vi "Test Read Speed.vi"(8 "error in (no error)":errorcluster) -> (0 "error out":errorcluster)   [LabVIEW 2016]
uses:
  LV to ITX/LV to ITX.lvclass
panel:
  in  "length":i32=250
  out "Numeric 3":i32
  out "Numeric 2":i32
  out "Numeric":i32
  out "read TDMS (ms/file)":u32
  out "read HDF5 (ms/file)":u32
  out "read ITX (ms/file)":u32
  in  "TDMS Path":path
  in  "HDF5 Path":path
  in  "ITX Path":path
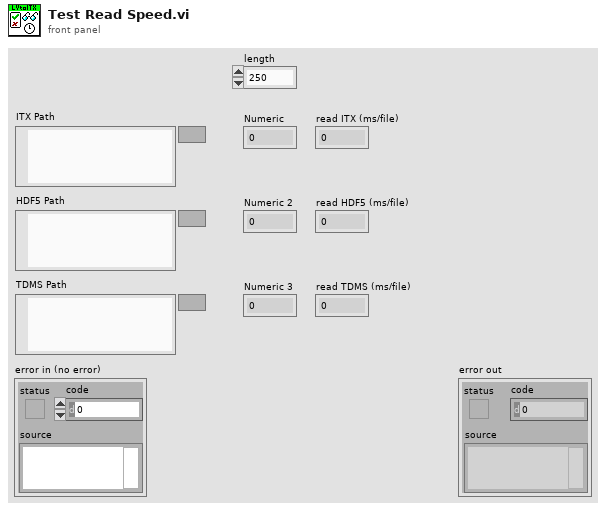
[diagram p1: front panel]
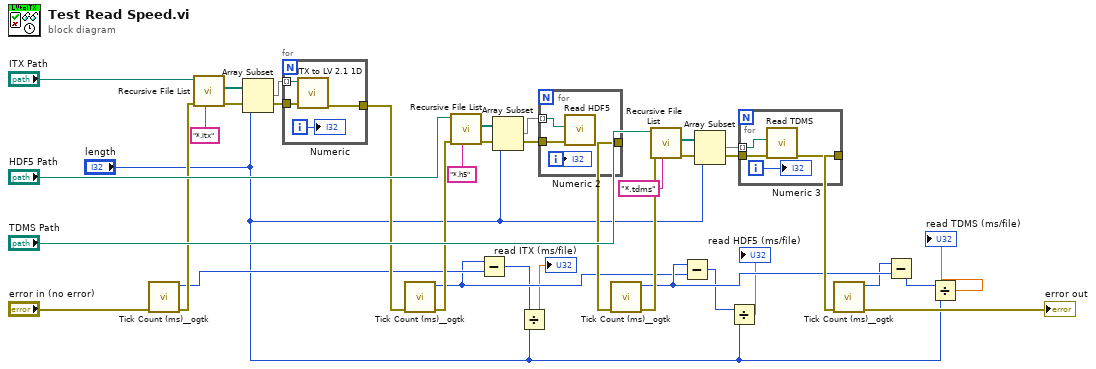
[diagram p0: block diagram]
diagram:
  n1 = call <userlib>:"Tick Count (ms)__ogtk.vi"("error in (no error)"="error in (no error)") -> ("error out"=w26:errorcluster, "millisecond timer value"=w15:u32)  [unwired: 9 in]
  n2 = call <vilib>:"Recursive File List.vi"("pattern"="*.itx", "error in (no error)"=w26, "Folder Path"="ITX Path") -> ("error out"=w9:errorcluster, "All Files in Dir"=w12:path[])  [unwired: 4 in, 3 out]
  n3 = Array Subset(array=w12, length="length") -> (w10:path[])  [unwired: 1 in]
  n4 = for {
    tunnel: w10 -> [w38] mode=indexing
    tunnel: [w37] -> w22
    tunnel: w9 -> [w36]
    i -> [w35]
    n5 = call "ITX to LV 2.1 1D.vi"("error in"=w36, "file (use dialog)"=w38) -> ("error out"=w37:errorcluster)  [unwired: 4 in, 5 out]
    "Numeric" <- w35
  }
  n6 = call <userlib>:"Tick Count (ms)__ogtk.vi"("error in (no error)"=w22) -> ("error out"=w21:errorcluster, "millisecond timer value"=w8:u32)  [unwired: 9 in]
  n7 = call <vilib>:"Recursive File List.vi"("pattern"="*.h5", "error in (no error)"=w21, "Folder Path"="HDF5 Path") -> ("error out"=w20:errorcluster, "All Files in Dir"=w29:path[])  [unwired: 4 in, 3 out]
  n8 = Subtract(x=w8, y=w15) -> (x-y=w7:u32)
  n9 = Array Subset(array=w29, length="length") -> (w24:path[])  [unwired: 1 in]
  n10 = Divide(x=w7, y="length") -> (x/y=→"read ITX (ms/file)":dbl)
  n11 = for {
    tunnel: w24 -> [w39] mode=indexing
    tunnel: w20 -> [w42]
    tunnel: [w41] -> w19
    i -> [w40]
    n12 = call "Read HDF5.vi"("error in (no error)"=w42, "path"=w39) -> ("error out"=w41:errorcluster)  [unwired: 4 in, 5 out]
    "Numeric 2" <- w40
  }
  n13 = call <userlib>:"Tick Count (ms)__ogtk.vi"("error in (no error)"=w19) -> ("error out"=w18:errorcluster, "millisecond timer value"=w14:u32)  [unwired: 9 in]
  n14 = call <vilib>:"Recursive File List.vi"("pattern"="*.tdms", "error in (no error)"=w18, "Folder Path"="TDMS Path") -> ("error out"=w17:errorcluster, "All Files in Dir"=w28:path[])  [unwired: 4 in, 3 out]
  n15 = Subtract(x=w14, y=w8) -> (x-y=w5:u32)
  n16 = Array Subset(array=w28, length="length") -> (w23:path[])  [unwired: 1 in]
  n17 = Divide(x=w5, y="length") -> (x/y=→"read HDF5 (ms/file)":dbl)
  n18 = for {
    tunnel: w23 -> [w46] mode=indexing
    tunnel: w17 -> [w45]
    tunnel: [w44] -> w16
    i -> [w43]
    n19 = call "Read TDMS.vi"("error in (no error)"=w45, "path"=w46) -> ("error out"=w44:errorcluster)  [unwired: 3 in, 6 out]
    "Numeric 3" <- w43
  }
  n20 = call <userlib>:"Tick Count (ms)__ogtk.vi"("error in (no error)"=w16) -> ("error out"=→"error out":errorcluster, "millisecond timer value"=w13:u32)  [unwired: 9 in]
  n21 = Subtract(x=w13, y=w14) -> (x-y=w3:u32)
  n22 = Divide(x=w3, y="length") -> (x/y=→"read TDMS (ms/file)":dbl)
